vi "main.vi"() -> ()   [LabVIEW 2020]
uses:
  <vilib>/express/express arith-compare/Formula/XNode/ExpressFormulaBlockNode.xnode
  <vilib>/Analysis/NI_AALBase.lvlib
panel:
  in  "?":T1(tab)
  in  "码元样本个数":i32=1000000
  in  "噪声方差":dbl=0.02
  out "最小误码率":dbl
  out "最佳判决门限":dbl
  in  "噪声方差":dbl=0.5
  out "误码率":dbl
  out "最佳判决门限时误码率随噪声方差的变化曲线":dbl[](graph)
  in  "码元样本个数":i32=1000000
  in  "观测次数":i32=5
  in  "噪声方差":dbl=0.5
  out "误码率":dbl
  out "第1种的误码率":dbl
  in  "噪声方差":dbl=0.5
  out "第2种的误码率":dbl
  in  "噪声方差":dbl=0.5
  out "方案一误码率":dbl
  out "方案二误码率":dbl
  out "最佳方案误码率":dbl
  # "5-1"
  # "输入控制"
  # "输出结果"
  # "输入控制"
  # "输出结果"
  # "5-2"
  # "码元样本个数\n 10000000"
  # "判决门限\n 0.5"
  # "5-3"
  # "输入控制"
  # "输出结果"
  # "码元样本个数\n 10000000"
  # "判决门限\n 0.5"
  # "输入控制"
  # "输出结果"
  # "5-4"
  # "码元样本个数\n 10000000"
  # "判决门限\n 0.5"
  # "观测次数\n 10"
  # "输入控制"
  # "输出结果"
  # "码元样本个数\n 10000000"
  # "判决门限\n 0.5"
  # "观测次数\n 10"
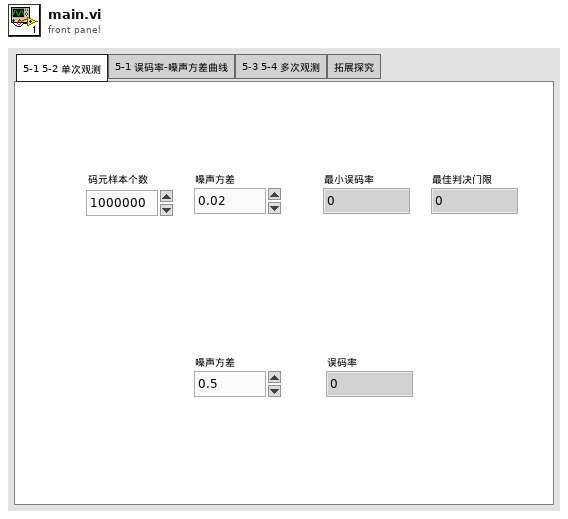
[diagram p1: front panel]
types:
  T1 = enum32{"5-1 5-2 单次观测", "5-1 误码率-噪声方差曲线", "5-3 5-4 多次观测", "拓展探究"}
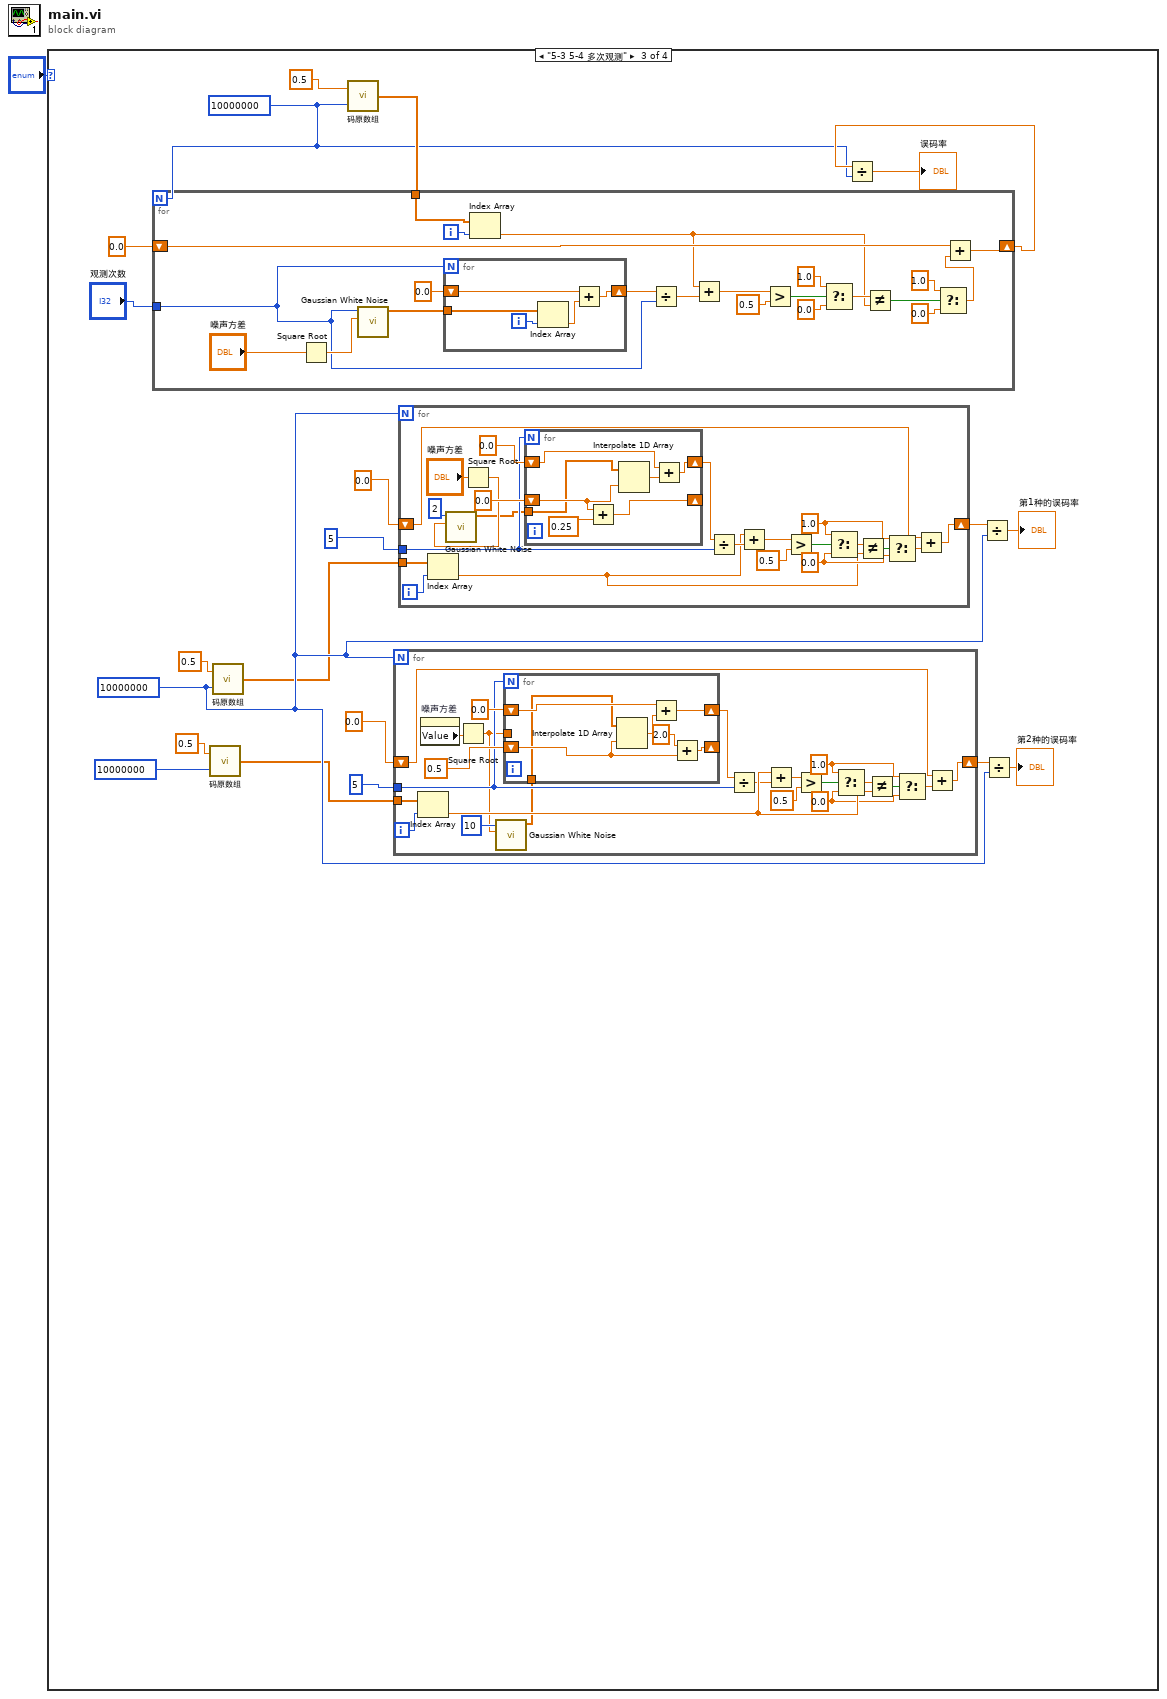
[diagram p0: block diagram]
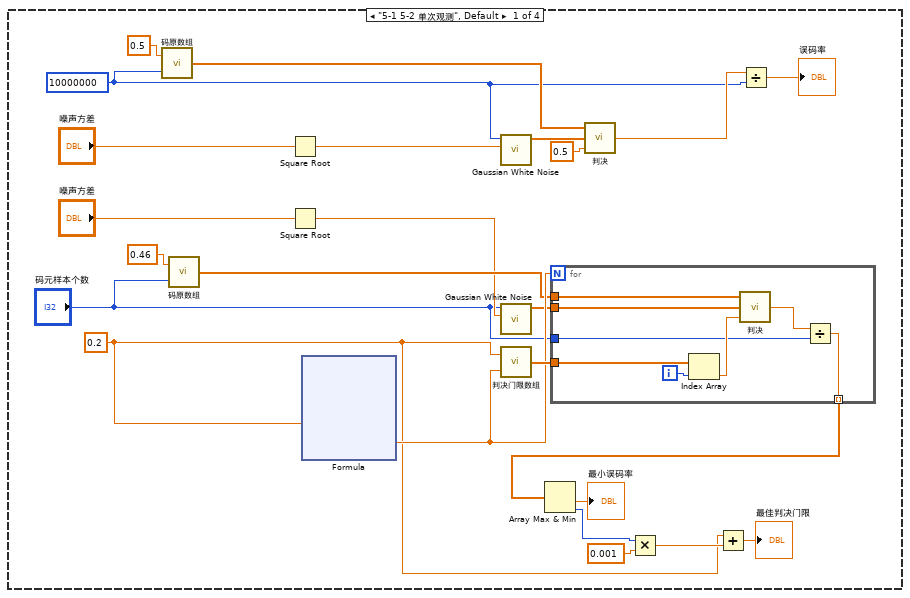
[diagram p2: hidden frame]
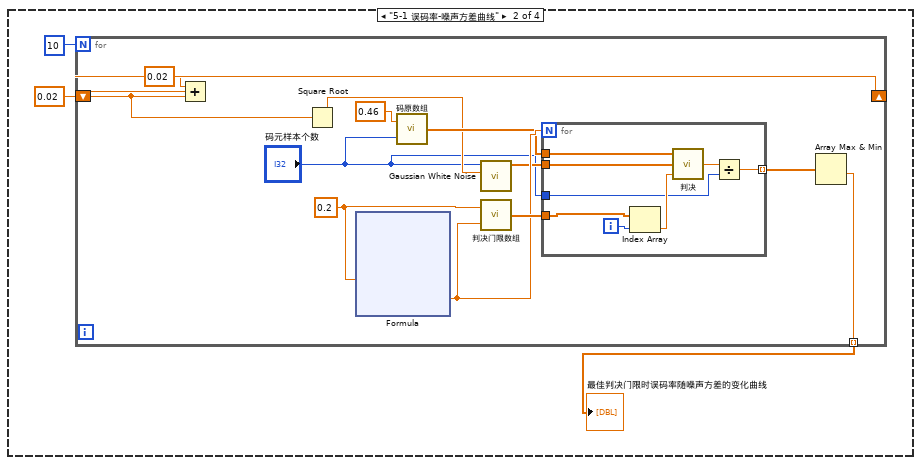
[diagram p3: hidden frame]
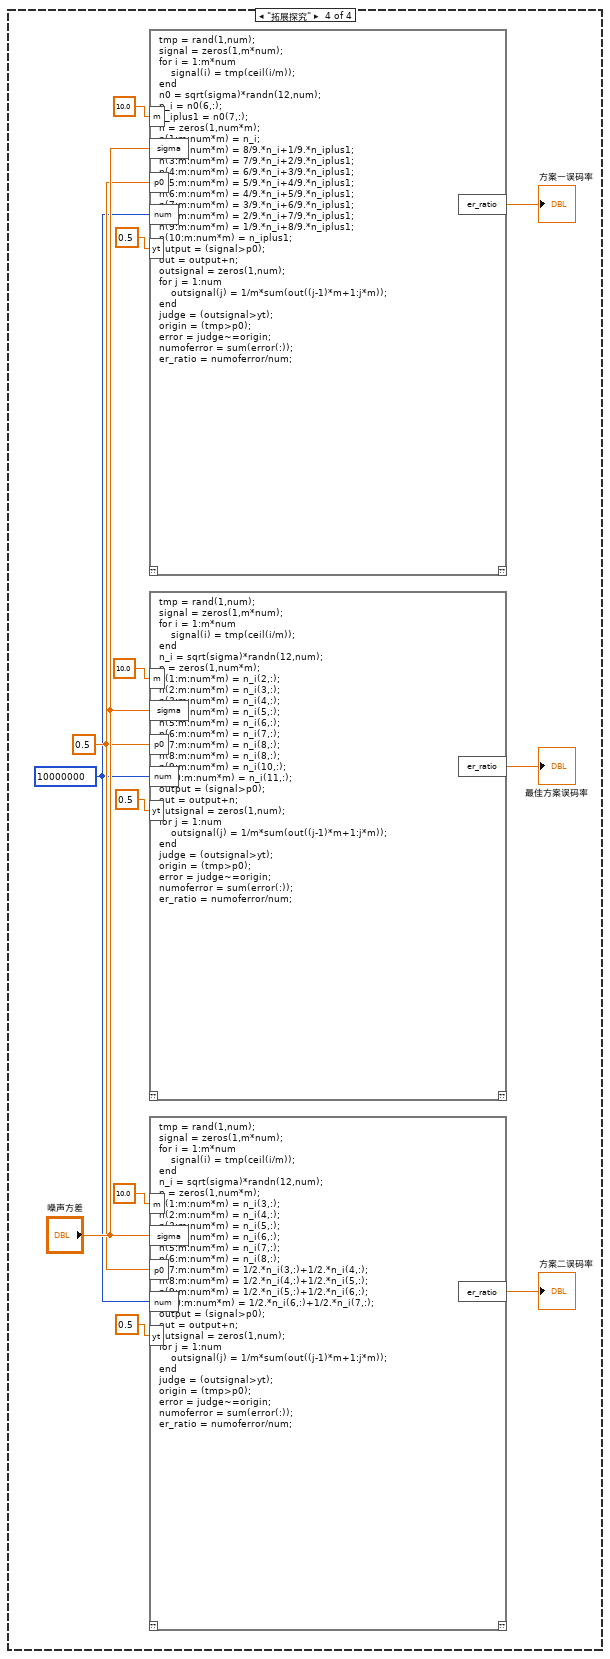
[diagram p4: hidden frame]
diagram:
  n1 = case shown="\"5-3 5-4 多次观测\"" "?" {
    frame "5-1 5-2 单次观测", Default {
      w4 = 10000000 ("码元样本个数 2")
      w15 = 0.2 ("t")
      n2 = call "码原数组.vi"("码元样本个数"=w4, "P(H0)"=0.5 ("y")) -> ("码元数组"=w8:dbl[])
      n3 = call "码原数组.vi"("码元样本个数"="码元样本个数", "P(H0)"=0.46 ("y")) -> ("码元数组"=w23:dbl[])
      n4 = Square Root(x="噪声方差") -> (sqrt(x)=w11:dbl)
      n5 = Square Root(x="噪声方差") -> (sqrt(x)=w22:dbl)
      n6 = xnode "Formula"("Start"=w15) -> ("Result"=w24:dbl)  [unwired: 1 in, 1 out]
      n7 = call <vilib>:"Gaussian White Noise.vi"("standard deviation"=w11, "samples"=w4) -> ("Gaussian noise pattern"=w7:dbl[])  [unwired: 8 in, 1 out]
      n8 = call <vilib>:"Gaussian White Noise.vi"("standard deviation"=w22, "samples"="码元样本个数") -> ("Gaussian noise pattern"=w19:dbl[])  [unwired: 8 in, 1 out]
      n9 = call "判决门限数组.vi"("尝试次数"=w24, "Start"=w15) -> ("判决门限数组"=w25:dbl[])
      n10 = for {
        N: w24 -> [_]
        tunnel: "码元样本个数" -> [w36]
        tunnel: w19 -> [w39]
        tunnel: w23 -> [w40]
        tunnel: w25 -> [w35]
        tunnel: [w34] -> w2 mode=indexing
        i -> [w41]
        n11 = Index Array(array=w35, index=w41) -> (element=w38:dbl)
        n12 = call "判决.vi"("判决门限"=w38, "噪声数组"=w39, "码元数组"=w40) -> ("错误计数"=w37:dbl)
        n13 = Divide(x=w37, y=w36) -> (x/y=w34:dbl)
      }
      n14 = Array Max & Min(array=w2) -> (min value=→"最小误码率":dbl, min index (indices)=w18:i32)  [unwired: 2 out]
      n15 = call "判决.vi"("判决门限"=0.5, "噪声数组"=w7, "码元数组"=w8) -> ("错误计数"=w9:dbl)
      n16 = Multiply(x=w18, y=0.001) -> (x*y=w17:dbl)
      n17 = Add(x=w15, y=w17) -> (x+y=→"最佳判决门限":dbl)
      n18 = Divide(x=w9, y=w4) -> (x/y=→"误码率":dbl)
    }
    frame "5-1 误码率-噪声方差曲线" {
      n19 = for {
        N: 10 -> [_]
        shift-right: [w48] -> _
        shift-left: 0.02 -> [w46]
        tunnel: [w45] -> w42 mode=indexing
        w51 = 0.2 ("t")
        n20 = Add(x=0.02, y=w46) -> (x+y=w48:dbl)
        n21 = Square Root(x=w46) -> (sqrt(x)=w54:dbl)
        n22 = xnode "Formula"("Start"=w51) -> ("Result"=w56:dbl)  [unwired: 1 in, 1 out]
        n23 = call "码原数组.vi"("码元样本个数"="码元样本个数", "P(H0)"=0.46 ("y")) -> ("码元数组"=w55:dbl[])
        n24 = call <vilib>:"Gaussian White Noise.vi"("standard deviation"=w54, "samples"="码元样本个数") -> ("Gaussian noise pattern"=w53:dbl[])  [unwired: 8 in, 1 out]
        n25 = call "判决门限数组.vi"("尝试次数"=w56, "Start"=w51) -> ("判决门限数组"=w57:dbl[])
        n26 = for {
          N: w56 -> [_]
          tunnel: "码元样本个数" -> [w67]
          tunnel: w53 -> [w70]
          tunnel: [w72] -> w52 mode=indexing
          tunnel: w55 -> [w71]
          tunnel: w57 -> [w66]
          i -> [w73]
          n27 = Index Array(array=w66, index=w73) -> (element=w69:dbl)
          n28 = call "判决.vi"("判决门限"=w69, "噪声数组"=w70, "码元数组"=w71) -> ("错误计数"=w68:dbl)
          n29 = Divide(x=w68, y=w67) -> (x/y=w72:dbl)
        }
        n30 = Array Max & Min(array=w52) -> (min value=w45:dbl)  [unwired: 3 out]
      }
      "最佳判决门限时误码率随噪声方差的变化曲线" <- w42
    }
    frame "5-3 5-4 多次观测" {
      w83 = 10000000 ("码元样本个数 2")
      w90 = 10000000 ("码元样本个数 2")
      n31 = call "码原数组.vi"("码元样本个数"=10000000 ("码元样本个数 2"), "P(H0)"=0.5 ("y")) -> ("码元数组"=w79:dbl[])
      n32 = call "码原数组.vi"("码元样本个数"=w83, "P(H0)"=0.5 ("y")) -> ("码元数组"=w78:dbl[])
      n33 = call "码原数组.vi"("码元样本个数"=w90, "P(H0)"=0.5 ("y")) -> ("码元数组"=w92:dbl[])
      n34 = for {
        N: w90 -> [_]
        shift-right: [w155] -> w91
        shift-left: 0.0 -> [w167]
        tunnel: w92 -> [w156]
        tunnel: "观测次数" -> [w153]
        i -> [w165]
        n35 = Square Root(x="噪声方差") -> (sqrt(x)=w160:dbl)
        n36 = call <vilib>:"Gaussian White Noise.vi"("standard deviation"=w160, "samples"=w153) -> ("Gaussian noise pattern"=w159:dbl[])  [unwired: 8 in, 1 out]
        n37 = for {
          N: w153 -> [_]
          shift-right: [w178] -> w158
          shift-left: 0.0 -> [w179]
          tunnel: w159 -> [w175]
          i -> [w177]
          n38 = Index Array(array=w175, index=w177) -> (element=w176:dbl)
          n39 = Add(x=w179, y=w176) -> (x+y=w178:dbl)
        }
        n40 = Index Array(array=w156, index=w165) -> (element=w164:dbl)
        n41 = Divide(x=w158, y=w153) -> (x/y=w157:dbl)
        n42 = Add(x=w164, y=w157) -> (x+y=w166:dbl)
        n43 = Greater?(x=w166, y=0.5) -> (0:w172:bool)
        n44 = Select(t=1.0, s=w172, f=0.0) -> (s? t:f=w171:dbl)
        n45 = Not Equal?(x=w171, y=w164) -> (x != y?=w170:bool)
        n46 = Select(t=1.0, s=w170, f=0.0) -> (s? t:f=w154:dbl)
        n47 = Add(x=w167, y=w154) -> (x+y=w155:dbl)
      }
      n48 = for {
        N: w83 -> [_]
        shift-right: [w111] -> w76
        shift-left: 0.0 -> [w112]
        tunnel: w79 -> [w107]
        tunnel: 5 ("观测次数 3") -> [w101]
        i -> [w109]
        w99 = 0.0
        w100 = 1.0
        n49 = Index Array(array=w107, index=w109) -> (element=w108:dbl)
        n50 = property on="噪声方差" class="DigNum (strict)"() -> ("Value"=w95:dbl)  [unwired: 2 in, 2 out]
        n51 = Square Root(x=w95) -> (sqrt(x)=w97:dbl)
        n52 = call <vilib>:"Gaussian White Noise.vi"("standard deviation"=w97, "samples"=10) -> ("Gaussian noise pattern"=w96:dbl[])  [unwired: 8 in, 1 out]
        n53 = for {
          N: w101 -> [_]
          tunnel: w97 -> [_]
          shift-right: [w123] -> _
          shift-left: 0.5 -> [w119]
          shift-right: [w121] -> w105
          shift-left: 0.0 -> [w122]
          tunnel: w96 -> [w117]
          n54 = Interpolate 1D Array(1:w119, 2:w117) -> (0:w120:dbl)
          n55 = Add(x=w122, y=w120) -> (x+y=w121:dbl)
          n56 = Add(x=2.0 ("y"), y=w119) -> (x+y=w123:dbl)
        }
        n57 = Divide(x=w105, y=w101) -> (x/y=w102:dbl)
        n58 = Add(x=w108, y=w102) -> (x+y=w110:dbl)
        n59 = Greater?(x=w110, y=0.5) -> (0:w116:bool)
        n60 = Select(t=w100, s=w116, f=w99) -> (s? t:f=w115:dbl)
        n61 = Not Equal?(x=w115, y=w108) -> (x != y?=w114:bool)
        n62 = Select(t=w100, s=w114, f=w99) -> (s? t:f=w113:dbl)
        n63 = Add(x=w112, y=w113) -> (x+y=w111:dbl)
      }
      n64 = for {
        N: w83 -> [_]
        shift-right: [w140] -> w88
        shift-left: 0.0 -> [w141]
        tunnel: w78 -> [w137]
        tunnel: 5 ("观测次数 2") -> [w130]
        i -> [w138]
        w128 = 0.0
        w129 = 1.0
        n65 = Index Array(array=w137, index=w138) -> (element=w127:dbl)
        n66 = Square Root(x="噪声方差") -> (sqrt(x)=w125:dbl)
        n67 = call <vilib>:"Gaussian White Noise.vi"("standard deviation"=w125, "samples"=2) -> ("Gaussian noise pattern"=w124:dbl[])  [unwired: 8 in, 1 out]
        n68 = for {
          N: w130 -> [_]
          shift-right: [w152] -> _
          shift-left: 0.0 -> [w150]
          shift-right: [w148] -> w135
          shift-left: 0.0 -> [w149]
          tunnel: w124 -> [w146]
          n69 = Add(x=w150, y=0.25) -> (x+y=w152:dbl)
          n70 = Interpolate 1D Array(1:w150, 2:w146) -> (0:w147:dbl)
          n71 = Add(x=w149, y=w147) -> (x+y=w148:dbl)
        }
        n72 = Divide(x=w135, y=w130) -> (x/y=w131:dbl)
        n73 = Add(x=w127, y=w131) -> (x+y=w139:dbl)
        n74 = Greater?(x=w139, y=0.5) -> (0:w145:bool)
        n75 = Select(t=w129, s=w145, f=w128) -> (s? t:f=w144:dbl)
        n76 = Not Equal?(x=w144, y=w127) -> (x != y?=w143:bool)
        n77 = Select(t=w129, s=w143, f=w128) -> (s? t:f=w142:dbl)
        n78 = Add(x=w141, y=w142) -> (x+y=w140:dbl)
      }
      n79 = Divide(x=w91, y=w90) -> (x/y=→"误码率":dbl)
      n80 = Divide(x=w88, y=w83) -> (x/y=→"第1种的误码率":dbl)
      n81 = Divide(x=w76, y=w83) -> (x/y=→"第2种的误码率":dbl)
    }
    frame "拓展探究" {
      w180 = 10000000
      w181 = 0.5
      n82 = script code="tmp = rand(1,num);\nsignal = zeros(1,m*num);\nfor i = 1:m*num\n    signal(i) = tmp(ceil(i/m));\nend\nn0 = sqrt(sigma)*randn(12,num);\nn_i = n0(6,:);\nn_iplus1 = n0(7,:);\nn = zeros(1,num*m);\nn(1:m:num*m) = n_i;\nn(2:m:num*m) = 8/9.*n_i+1/9.*n_iplus1;\nn(3:m:num*m) = 7/9.*n_i+2/9.*n_iplus1;\nn(4:m:num*m) = 6/9.*n_i+3/9.*n_iplus1;\nn(5:m:num*m) = 5/9.*n_i+4/9.*n_iplus1;\nn(6:m:num*m) = 4/9.*n_i+5/9.*n_iplus1;\nn(7:m:num*m) = 3/9.*n_i+6/9.*n_iplus1;\nn(8:m:num*m) = 2/9.*n_i+7/9.*n_iplus1;\nn(9:m:num*m) = 1/9.*n_i+8/9.*n_iplus1;\nn(10:m:num*m) = n_iplus1;\noutput = (signal>p0);\nout = output+n;\noutsignal = zeros(1,num);\nfor j = 1:num\n    outsignal(j) = 1/m*sum(out((j-1)*m+1:j*m));\nend\njudge = (outsignal>yt);\norigin = (tmp>p0);\nerror = judge~=origin;\nnumoferror = sum(error(:));\ner_ratio = numoferror/num;"("p0"=w181, "num"=w180, "sigma"="噪声方差", "yt"=0.5 ("Real"), "m"=10.0 ("Real")) -> ("er_ratio"=→"方案一误码率":dbl)  [unwired: 1 in, 1 out]
      n83 = script code="tmp = rand(1,num);\nsignal = zeros(1,m*num);\nfor i = 1:m*num\n    signal(i) = tmp(ceil(i/m));\nend\nn_i = sqrt(sigma)*randn(12,num);\nn = zeros(1,num*m);\nn(1:m:num*m) = n_i(2,:);\nn(2:m:num*m) = n_i(3,:);\nn(3:m:num*m) = n_i(4,:);\nn(4:m:num*m) = n_i(5,:);\nn(5:m:num*m) = n_i(6,:);\nn(6:m:num*m) = n_i(7,:);\nn(7:m:num*m) = n_i(8,:);\nn(8:m:num*m) = n_i(8,:);\nn(9:m:num*m) = n_i(10,:);\nn(10:m:num*m) = n_i(11,:);\noutput = (signal>p0);\nout = output+n;\noutsignal = zeros(1,num);\nfor j = 1:num\n    outsignal(j) = 1/m*sum(out((j-1)*m+1:j*m));\nend\njudge = (outsignal>yt);\norigin = (tmp>p0);\nerror = judge~=origin;\nnumoferror = sum(error(:));\ner_ratio = numoferror/num;"("p0"=w181, "num"=w180, "sigma"="噪声方差", "yt"=0.5 ("Real"), "m"=10.0 ("Real")) -> ("er_ratio"=→"最佳方案误码率":dbl)  [unwired: 1 in, 1 out]
      n84 = script code="tmp = rand(1,num);\nsignal = zeros(1,m*num);\nfor i = 1:m*num\n    signal(i) = tmp(ceil(i/m));\nend\nn_i = sqrt(sigma)*randn(12,num);\nn = zeros(1,num*m);\nn(1:m:num*m) = n_i(3,:);\nn(2:m:num*m) = n_i(4,:);\nn(3:m:num*m) = n_i(5,:);\nn(4:m:num*m) = n_i(6,:);\nn(5:m:num*m) = n_i(7,:);\nn(6:m:num*m) = n_i(8,:);\nn(7:m:num*m) = 1/2.*n_i(3,:)+1/2.*n_i(4,:);\nn(8:m:num*m) = 1/2.*n_i(4,:)+1/2.*n_i(5,:);\nn(9:m:num*m) = 1/2.*n_i(5,:)+1/2.*n_i(6,:);\nn(10:m:num*m) = 1/2.*n_i(6,:)+1/2.*n_i(7,:);\noutput = (signal>p0);\nout = output+n;\noutsignal = zeros(1,num);\nfor j = 1:num\n    outsignal(j) = 1/m*sum(out((j-1)*m+1:j*m));\nend\njudge = (outsignal>yt);\norigin = (tmp>p0);\nerror = judge~=origin;\nnumoferror = sum(error(:));\ner_ratio = numoferror/num;"("p0"=w181, "num"=w180, "sigma"="噪声方差", "yt"=0.5 ("Real"), "m"=10.0 ("Real")) -> ("er_ratio"=→"方案二误码率":dbl)  [unwired: 1 in, 1 out]
    }
  }
